vi "Get RIO Image.vi"() -> ()   [LabVIEW 2019]
uses:
  <vilib>/nisyscfg/nisyscfg.lvlib
panel:
  out "error out":errorcluster
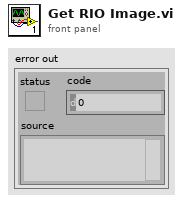
[diagram p1: front panel]
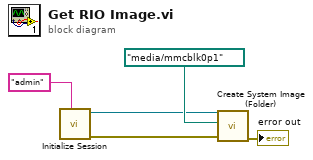
[diagram p0: block diagram]
diagram:
  n1 = call <vilib>:"Initialize Session.vi"("User Name"="admin") -> ("error out"=w2:errorcluster, "Session out"=w3:refnum<k21>)  [unwired: 9 in]
  n2 = call <vilib>:"Create System Image (Folder).vi"("error in (no error)"=w2, "Destination Folder"=path "/media/mmcblk0p1", "Session in"=w3) -> ("error out"=→"error out":errorcluster)  [unwired: 6 in, 2 out]
